vi "sendClusterfromServer.vi"() -> ()   [LabVIEW 2019]
panel:
  in  "stop":bool
  in  "Cluster":T1
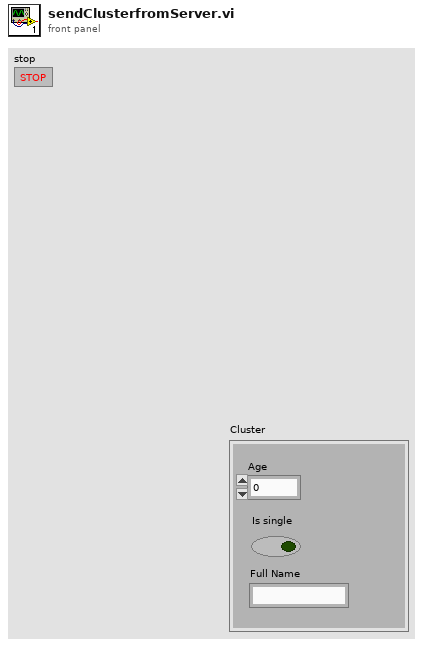
[diagram p1: front panel]
types:
  T1 = cluster{"Age":dbl, "Is single":bool, "Full Name":string}
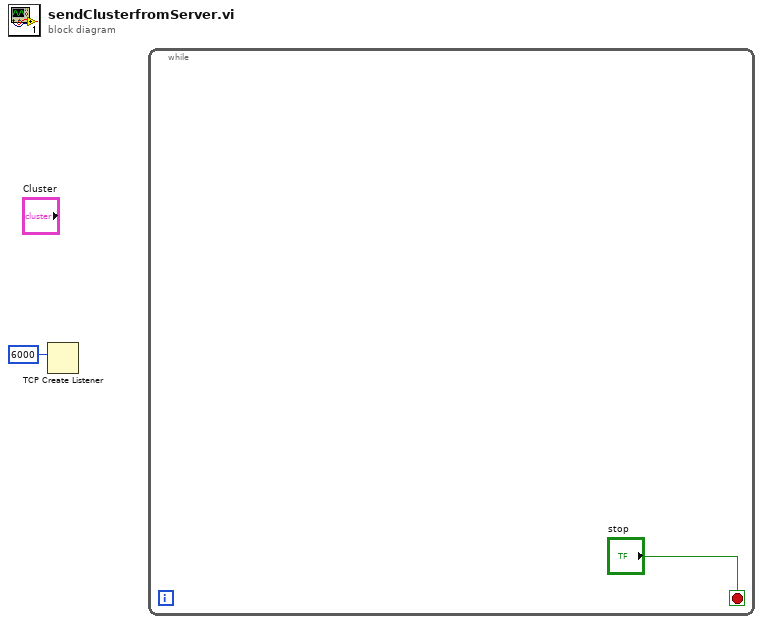
[diagram p0: block diagram]
diagram:
  n1 = TCP Create Listener(10:u16 6000 ("port")) -> ()  [unwired: 4 in, 3 out]
  n2 = while {
    stop <- "stop" stop-if-true
  }
